vi "init.vi"(8 "error in":errorcluster, 10 "TBM module configuration in":refnum<class "TBM module configuration.lvclass">, 11 "TDMS datalogger runtime in":refnum<class "TDMS datalogger runtime.lvclass">) -> (0 "error out":errorcluster, 1 "data allocations":T1, 2 "execution settings":T4, 3 "TDMS datalogger runtime out":refnum<class "TDMS datalogger runtime.lvclass">)   [LabVIEW 2013, in "TDMS datalogger runtime.lvclass"]
doc: "Provides an interface for initializing a module at runtime. While this interface performs no operations, a child should provide an override which may open any necessary references or sessions, allocate necessary memory, and perform any final configuration validataion before providing the full configuration <b>execution data</b> to the calling process."
uses:
  TDMS datalogger runtime.lvclass
  <vilib>/NI/Tag Bus Module Framework/channel/TBM channel.lvclass
  <vilib>/NI/Tag Bus Module Framework/runtime/TBM module execution interface.lvclass
  configuration/TDMS datalogger configuration.lvclass
  <vilib>/NI/Tag Bus Module Framework/runtime/execution settings.ctl
  <vilib>/NI/Tag Bus/dictionary/data dictionary.lvclass
  control enum.ctl
  <vilib>/NI/Tag Bus/table/data table.ctl
  <vilib>/NI/Tag Bus/table/data table.lvlib
  message to background process.ctl
  response enum.ctl
  response from background process.ctl
  <vilib>/NI/Tag Bus Module Framework/module configuration/TBM module configuration.lvclass
  <vilib>/NI/Tag Bus Module Framework/channel/data tables.ctl
  <vilib>/NI/Tag Bus/dictionary table pair.ctl
  <vilib>/NI/Tag Bus/tag bus.lvlib
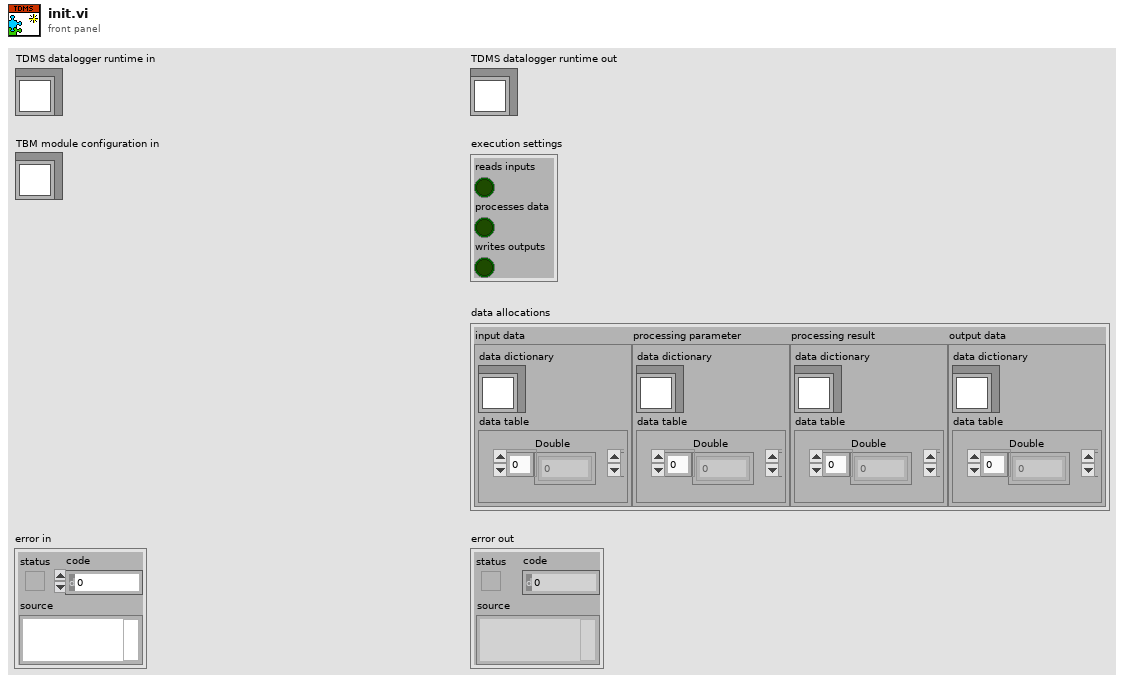
[diagram p1: front panel]
types:
  T1 = typedef "TBM channel.lvclass/data tables.ctl" = cluster{"input data":T2, "processing parameter":T2, "processing result":T2, "output data":T2}
  T2 = typedef "tag bus.lvlib/dictionary table pair.ctl" = cluster{"data dictionary":refnum<class "data dictionary.lvclass">, "data table":T3}
  T3 = typedef "tag bus.lvlib/data table.lvlib/data table.ctl" = cluster{"Double":dbl[], "Single":sgl[], "I64":i64[], "I32":i32[], "I16":i16[], "I8":i8[], "U64":u64[], "U32":u32[], "U16":u16[], "U8":u8[], "Boolean":bool[], "String":string[], "Array of Double":cluster{"DBL Array":dbl[]}[], "Array of Single":cluster{"SGL Array":sgl[]}[], "Array of I64":cluster{"I64 Array":i64[]}[], "Array of I32":cluster{"I32 Array":i32[]}[], "Array of I16":cluster{"I16 Array":i16[]}[], "Array of I8":cluster{"I8 Array":i8[]}[], "Array of U64":cluster{"U64 Array":u64[]}[], "Array of U32":cluster{"U32 Array":u32[]}[], "Array of U16":cluster{"U16 Array":u16[]}[], "Array of U8":cluster{"U8 Array":u8[]}[], "Array of Boolean":cluster{"Boolean Array":bool[]}[], "Array of String":cluster{"String Array":string[]}[]}
  T4 = typedef "TBM module execution interface.lvclass/execution settings.ctl" = cluster{"reads inputs":bool, "processes data":bool, "writes outputs":bool}
  T5 = cluster{"read mode":enum16{"polling", "blocking"}, "write mode":enum16{"polling", "blocking"}}
  T6 = typedef "TDMS datalogger runtime.lvclass/response from background process.ctl" = cluster{"response enum":T7, "datapack":refnum<data-value>, "error code":i32}
  T7 = typedef "TDMS datalogger runtime.lvclass/response enum.ctl" = enum16{"exit", "return buffer", "error"}
  T8 = typedef "TDMS datalogger runtime.lvclass/message to background process.ctl" = cluster{"control enum":T9, "datapack":refnum<data-value>, "Time Stamp":timestamp}
  T9 = typedef "TDMS datalogger runtime.lvclass/control enum.ctl" = enum16{"exit", "output data"}
  T10 = typedef "tag bus.lvlib/tag descriptor.lvclass/Data Type.ctl" = enum16{"Double", "Single", "I64", "I32", "I16", "I8", "U64", "U32", "U16", "U8", "Boolean", "String", "Array of Double", "Array of Single", "Array of I64", "Array of I32", "Array of I16", "Array of I8", "Array of U64", "Array of U32", "Array of U16", "Array of U8", "Array of Boolean", "Array of String"}
  T11 = typedef "tag bus.lvlib/data dictionary.lvclass/full data dictionary.ctl" = cluster{"Double":string[], "Single":string[], "I64":string[], "I32":string[], "I16":string[], "I8":string[], "U64":string[], "U32":string[], "U16":string[], "U8":string[], "Boolean":string[], "String":string[], "Array of Double":string[], "Array of Single":string[], "Array of I64":string[], "Array of I32":string[], "Array of I16":string[], "Array of I8":string[], "Array of U64":string[], "Array of U32":string[], "Array of U16":string[], "Array of U8":string[], "Array of Boolean":string[], "Array of String":string[]}
  T12 = typedef "tag bus.lvlib/data table.lvlib/allocation specification.ctl" = cluster{"data type":T10, "size":i32}
  T13 = typedef "TDMS datalogger runtime.lvclass/data cache.ctl" = cluster{"timestamps":timestamp[], "Double":dbl[][], "Single":sgl[][], "I64":i64[][], "I32":i32[][], "I16":i16[][], "I8":i8[][], "U64":u64[][], "U32":u32[][], "U16":u16[][], "U8":u8[][], "Boolean":bool[][]}
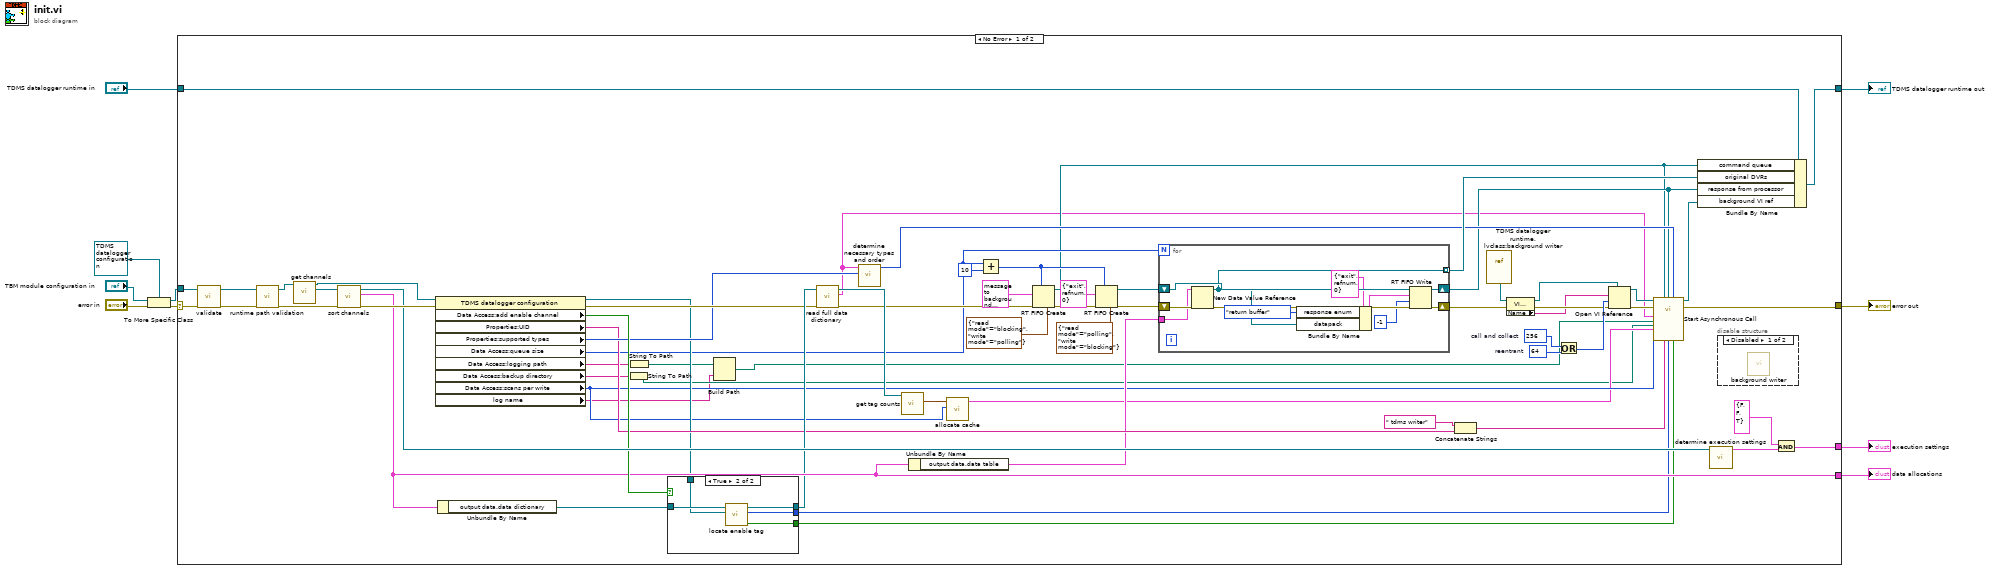
[diagram p0: block diagram]
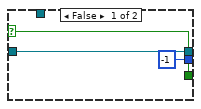
[diagram p2: hidden frame]
diagram:
  n1 = To More Specific Class(target class=refnum<class "TDMS datalogger configuration.lvclass"> refnum ("Synchronous module configuration"), reference="TBM module configuration in", error in="error in") -> (specific class reference=w9:refnum<class "TDMS datalogger configuration.lvclass">, error out=w10:errorcluster)
  n2 = case shown="No Error" w10 {
    selector: w10 -> [w72 w96]
    tunnel: w9 -> [w71 _]
    tunnel: "TDMS datalogger runtime in" -> [w70 w97]
    tunnel: [w69 w97] -> w4
    tunnel: [w58 w96] -> w3
    tunnel: [w55 _] -> w1
    tunnel: [w68 _] -> w2
    frame No Error {
      w63 = 64  # reentrant
      w62 = 256  # call and collect
      n3 = call-dynamic "validate.vi"("error in"=w72, "TDMS datalogger configuration in"=w71) -> ("error out"=w73:errorcluster, "TDMS datalogger configuration out"=w46:refnum<class "TDMS datalogger configuration.lvclass">)  [unwired: 8 in]
      n4 = call "runtime path validation.vi"("error in"=w73, "TDMS datalogger configuration in"=w46) -> ("error out"=w47:errorcluster, "TDMS datalogger configuration out"=w45:refnum<class "TDMS datalogger configuration.lvclass">)  [unwired: 8 in]
      n5 = call-dynamic "get channels.vi"("module configuration in"=w45) -> ("channels"=w43:refnum<class "TBM channel.lvclass">[], "module configuration out"=w44:refnum<class "TDMS datalogger configuration.lvclass">)  [unwired: 9 in]
      n6 = call <vilib>:"sort channels.vi"("error in"=w47, "channels in"=w43) -> ("error out"=w76:errorcluster, "data allocations"=w55:T1, "channels out"=w74:refnum<class "TBM channel.lvclass">[])  [unwired: 7 in]
      n7 = property class="TDMS datalogger configuration"(reference=w44, error in=w76) -> (reference out=w39:refnum<class "TDMS datalogger configuration.lvclass">, error out=w51:errorcluster, "Data Access:add enable channel"=w56:bool, "Properties:UID"=w49:string, "Properties:supported types"=w50:T10[], "Data Access:queue size"=w31:u16, "Data Access:logging path"=w16:string, "Data Access:backup directory"=w15:string, "Data Access:scans per write"=w22:u16, "log name"=w13:string)
      n8 = Unbundle By Name(w55) -> ("output data.data dictionary"=w57:refnum<class "data dictionary.lvclass">)
      n9 = String To Path(string=w15) -> (path=w14:path)
      n10 = String To Path(string=w16) -> (path=w12:path)
      n11 = case shown="True" w56 {
        selector: w56 -> [w79 _]
        tunnel: w57 -> [w78 w84]
        tunnel: [w78 w83] -> w53
        tunnel: [w79 w81] -> w25
        tunnel: [-1 ("index") w82] -> w24
        tunnel: w39 -> [_ w80]
        frame False {
        }
        frame True {
          n12 = call "locate enable tag.vi"("TDMS datalogger configuration"=w80, "data dictionary in"=w84) -> ("found?"=w81:bool, "index"=w82:i32, "data dictionary out"=w83:refnum<class "data dictionary.lvclass">)  [unwired: 7 in]
        }
      }
      n13 = Build Path(base path=w12, name or relative path=w13) -> (appended path=w11:path)
      n14 = call <vilib>:"read full data dictionary.vi"("error in"=w51, "data dictionary in"=w53) -> ("error out"=w41:errorcluster, "dictionary"=w17:T11, "data dictionary out"=w52:refnum<class "data dictionary.lvclass">)  [unwired: 7 in]
      n15 = call "determine necessary types and order.vi"("supported types"=w50, "dictionary"=w17) -> ("output type order"=w20:T10[])  [unwired: 9 in]
      n16 = call <vilib>:"get tag counts.vi"("data dictionary in"=w52) -> ("counts"=w66:T12[])  [unwired: 9 in, 1 out]
      n17 = Unbundle By Name(w55) -> ("output data.data table"=w42:T3)
      n18 = call "allocate cache.vi"("scans per write"=w22, "counts"=w66) -> ("cache allocation"=w21:T13)  [unwired: 9 in]
      n19 = Add(x=w31, y=u16 10) -> (x+y=w29:u16)
      n20 = RT FIFO Create(1:T8 {"control enum"=enum."exit", "datapack"=refnum, "Time Stamp"=timestamp(0 s since 1904-01-01)} ("message"), 3:w41, 4:w29, 7:T5 {"read mode"=enum."blocking", "write mode"=enum."polling"} ("r/w modes (polling,polling)")) -> (8:w18:refnum<k33>, 11:w40:errorcluster)  [unwired: 4 in, 1 out]
      n21 = RT FIFO Create(1:T6 {"response enum"=enum."exit", "datapack"=refnum, "error code"=0} ("message"), 3:w40, 4:w29, 7:T5 {"read mode"=enum."polling", "write mode"=enum."blocking"} ("r/w modes (polling,polling)")) -> (8:w32:refnum<k33>, 11:w36:errorcluster)  [unwired: 4 in, 1 out]
      n22 = for {
        N: w31 -> [_]
        shift-right: [w92] -> w59
        shift-left: w36 -> [w95]
        tunnel: w42 -> [w94]
        tunnel: [w86] -> w33 mode=indexing
        shift-right: [w91] -> w19
        shift-left: w32 -> [w90]
        n23 = New Data Value Reference(data value=w94, error in=w95) -> (data value reference=w86:refnum<data-value>, error out=w93:errorcluster)
        n24 = Bundle By Name(cluster=T6 {"response enum"=enum."exit", "datapack"=refnum, "error code"=0} ("element"), "response enum"=response_enum."return buffer", "datapack"=w86) -> (w87:T6)
        n25 = RT FIFO Write(0:w90, 1:w87, 2:-1 ("timeout in ms (0)"), 3:w93) -> (8:w91:refnum<k33>, 11:w92:errorcluster)  [unwired: 1 in, 2 out]
      }
      n26 = Concatenate Strings(" tdms writer" ("string"), w49) -> (w23:string)
      n27 = vi-ref "TDMS datalogger runtime.lvclass:background writer.vi"() -> (w28:refnum<vi>)
      n28 = property class="VI (strict)"(reference=w28, error in=w59) -> (reference out=w27:refnum<vi>, error out=w61:errorcluster, "Name"=w60:string)
      n29 = Or(x=w62, y=w63) -> (x .or. y?=w64:i32)
      n30 = Open VI Reference(type specifier VI Refnum (for type only)=w27, vi path=w60, options=w64, error in (no error)=w61) -> (vi reference=w26:refnum<vi>, error out=w65:errorcluster)  [unwired: 2 in]
      n31 = call-by-ref "Start Asynchronous Call"(reference=w26, error in=w65, "dictionary"=w17, "command queue"=w18, "response from processor"=w19, "output type order"=w20, "logging path"=w11, "backup directory"=w14, "cache allocation"=w21, "scans per write"=w22, "group name"=w23, "enable channel (bool)"=w24, "has enable channel"=w25) -> (reference out=w54:refnum<vi>, error out=w58:errorcluster)  [unwired: 4 in, 1 out]
      n32 = Bundle By Name(cluster=w70, "command queue"=w18, "original DVRs"=w33, "response from processor"=w19, "background VI ref"=w54) -> (w69:refnum<class "TDMS datalogger runtime.lvclass">)
      n33 = call <vilib>:"determine execution settings.vi"("channels"=w74) -> ("execution settings"=w75:T4)  [unwired: 10 in]
      n34 = disable-structure shown="Disabled" {
        frame Disabled {
          n35 = call "background writer.vi"() -> ()  [unwired: 15 in, 1 out]
        }
        frame Enabled {
        }
      }
      n36 = And(x=T4 {"reads inputs"=FALSE, "processes data"=FALSE, "writes outputs"=TRUE}, y=w75) -> (x .and. y?=w68:T4)
    }
    frame Error {
    }
  }
  "error out" <- w3
  "TDMS datalogger runtime out" <- w4
  "execution settings" <- w2
  "data allocations" <- w1
